vi "LabVIEW host computer v2.0.vi"() -> ()   [LabVIEW 2015]
uses:
  <vilib>/Instr/_visa.llb/VISA Configure Serial Port (Instr).vi
panel:
  out "CH1/CH2":dbl(graph)
  in  "选项卡控件":enum32{"串口配置 ", "数据显示"}(tab)
  in  "VISA resource name":refnum<visa-resource-name> caption="选择串口"
  in  "baud rate (9600)":u32=9600 caption="波特率"
  out "CH1 Power":dbl
  out "?":string
  out "CH2 Power":dbl
  out "?":string
  out "CH1/CH2":dbl format="%#_3g"
  out "当前时间":string
  out "CH2 Power":dbl(graph)
  out "CH1 Power":dbl(graph)
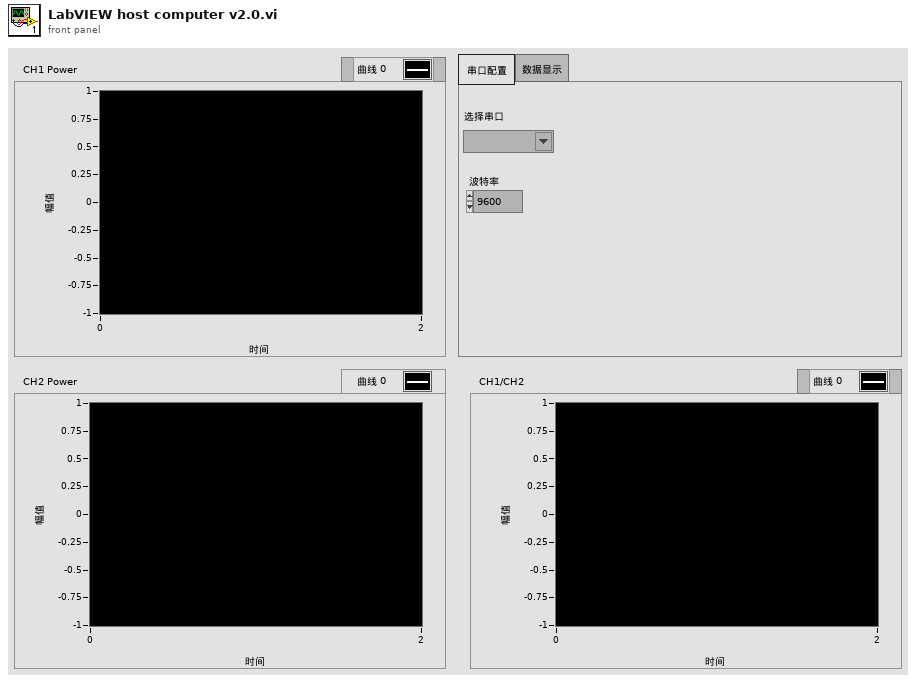
[diagram p1: front panel]
types:
  T1 = enum16{"open", "replace", "create", "open or create", "replace or create", "replace or create with confirmation"}
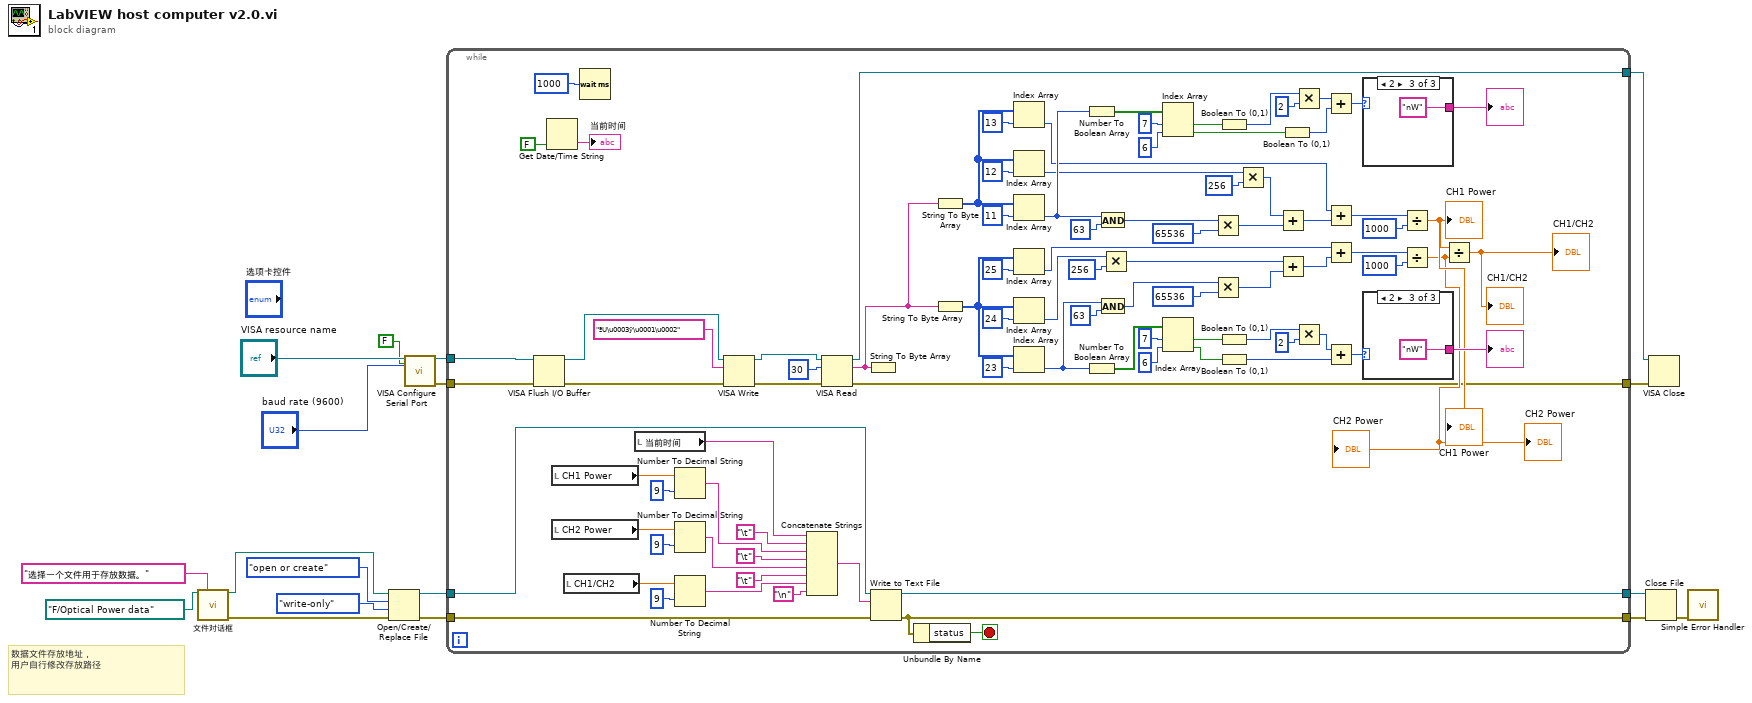
[diagram p0: block diagram]
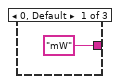
[diagram p2: hidden frame]
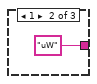
[diagram p3: hidden frame]
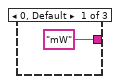
[diagram p4: hidden frame]
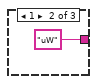
[diagram p5: hidden frame]
diagram:
  # "数据文件存放地址，\n用户自行修改存放路径"
  n1 = call "文件对话框"("start path"=path "F:/Optical Power data", "prompt"="选择一个文件用于存放数据。") -> ("selected path"=w9:path, "error out"=w8:errorcluster)  [unwired: 10 in, 2 out]
  n2 = Open/Create/Replace File(file path (use dialog)=w9, error in=w8, operation (0:open)=T1."open or create" ("操作(0:open)"), access (0:read/write)=enum16{"read/write", "read-only", "write-only"}."write-only" ("权限(0:read/write)")) -> (refnum out=w4:refnum<file>, error out=w5:errorcluster)  [unwired: 2 in, 1 out]
  n3 = call-poly "VISA Configure Serial Port"("VISA resource name"="VISA resource name", "Enable Termination\nChar (T)"=FALSE ("Enable Termination\nChar (T)"), "baud rate (9600)"="baud rate (9600)") -> ("VISA resource name out"=w15:refnum<visa-resource-name>, "error out"=w14:errorcluster)  [unwired: 11 in]
  n4 = while {
    tunnel: w15 -> [w48]
    tunnel: w14 -> [w47]
    tunnel: [w46] -> w13
    tunnel: [w43] -> w12
    tunnel: w5 -> [w41]
    tunnel: w4 -> [w40]
    tunnel: [w31] -> w2
    tunnel: [w33] -> w1
    stop <- w30 stop-if-true
    n5 = VISA Flush I/O Buffer(VISA resource name=w48, error in (no error)=w47) -> (VISA resource name out=w78:refnum<visa-resource-name>, error out=w77:errorcluster)  [unwired: 1 in]
    n6 = Get Date/Time String(want seconds? (F)=FALSE ("需要秒？(F)")) -> (time string=→"当前时间":string)  [unwired: 2 in, 1 out]
    n7 = local read "CH1 Power"() -> (w26:dbl)
    n8 = local read "CH2 Power"() -> (w25:dbl)
    n9 = local read "CH1/CH2"() -> (w24:dbl)
    n10 = Wait (ms)(milliseconds to wait=u32 1000 ("等待时间（毫秒）")) -> ()  [unwired: 1 out]
    n11 = local read "当前时间"() -> (w36:string)
    n12 = Number To Decimal String(number=w26, width (-)=i16 9 ("宽度(-)")) -> (decimal integer string=w23:string)
    n13 = Number To Decimal String(number=w25, width (-)=i16 9 ("宽度(-)")) -> (decimal integer string=w22:string)
    n14 = Number To Decimal String(number=w24, width (-)=i16 9 ("宽度(-)")) -> (decimal integer string=w19:string)
    n15 = VISA Write(VISA resource name=w78, write buffer="ªU\u0003ÿ\u0001\u0002" ("写入缓冲区"), error in (no error)=w77) -> (VISA resource name out=w108:refnum<visa-resource-name>, error out=w107:errorcluster)  [unwired: 1 out]
    n16 = Concatenate Strings(w36, "\t", w23, "\t", w22, "\t", w19, "\n") -> (w32:string)
    n17 = VISA Read(VISA resource name=w108, byte count=u32 30 ("字节总数"), error in (no error)=w107) -> (VISA resource name out=w46:refnum<visa-resource-name>, read buffer=w49:string, error out=w43:errorcluster)  [unwired: 1 out]
    n18 = String To Byte Array(string=w49) -> ()  [unwired: 1 out]
    n19 = Write to Text File(file (use dialog)=w40, text=w32, error in=w41) -> (refnum out=w33:refnum<file>, error out=w31:errorcluster)  [unwired: 1 in, 1 out]
    n20 = Unbundle By Name(w31) -> ("status"=w30:bool)
    n21 = String To Byte Array(string=w49) -> (unsigned byte array=w104:u8[])
    n22 = String To Byte Array(string=w49) -> (unsigned byte array=w75:u8[])
    n23 = Index Array(array=w104, index=13) -> (element=w89:u8)
    n24 = Index Array(array=w104, index=12) -> (element=w95:u8)
    n25 = Index Array(array=w104, index=11) -> (element=w101:u8)
    n26 = Index Array(array=w75, index=25) -> (element=w60:u8)
    n27 = Index Array(array=w75, index=24) -> (element=w66:u8)
    n28 = Index Array(array=w75, index=23) -> (element=w72:u8)
    n29 = Number To Boolean Array(number=w101) -> (Boolean array=w102:bool[])
    n30 = Number To Boolean Array(number=w72) -> (Boolean array=w73:bool[])
    n31 = And(x=w101, y=63) -> (x .and. y?=w93:i32)
    n32 = And(x=w72, y=63) -> (x .and. y?=w64:i32)
    n33 = Multiply(x=w66, y=u32 256) -> (x*y=w68:u32)
    n34 = Index Array(array=w102, index #1=7 ("index"), index #2=6 ("索引")) -> (element #1=w87:bool, element #2=w85:bool)
    n35 = Index Array(array=w73, index #1=7 ("index"), index #2=6 ("索引")) -> (element #1=w58:bool, element #2=w56:bool)
    n36 = Multiply(x=w93, y=u32 65536) -> (x*y=w98:u32)
    n37 = Multiply(x=w64, y=u32 65536) -> (x*y=w69:u32)
    n38 = Boolean To (0,1)(Boolean=w87) -> (0, 1=w86:i16)
    n39 = Boolean To (0,1)(Boolean=w58) -> (0, 1=w57:i16)
    n40 = Boolean To (0,1)(Boolean=w56) -> (0, 1=w53:i16)
    n41 = Multiply(x=w95, y=u32 256) -> (x*y=w97:u32)
    n42 = Add(x=w97, y=w98) -> (x+y=w99:u32)
    n43 = Add(x=w68, y=w69) -> (x+y=w70:u32)
    n44 = Boolean To (0,1)(Boolean=w85) -> (0, 1=w82:i16)
    n45 = Multiply(x=w86, y=2 ("index")) -> (x*y=w83:i32)
    n46 = Multiply(x=w57, y=2 ("index")) -> (x*y=w54:i32)
    n47 = Add(x=w83, y=w82) -> (x+y=w81:i32)
    n48 = Add(x=w89, y=w99) -> (x+y=w80:u32)
    n49 = Add(x=w60, y=w70) -> (x+y=w51:u32)
    n50 = Add(x=w54, y=w53) -> (x+y=w52:i32)
    n51 = case shown="2" w81 {
      tunnel: ["mW" "uW" "nW"] -> w79
      frame 0, Default {
      }
      frame 1 {
      }
      frame 2 {
      }
    }
    "?" <- w79
    n52 = case shown="2" w52 {
      tunnel: ["mW" "uW" "nW"] -> w50
      frame 0, Default {
      }
      frame 1 {
      }
      frame 2 {
      }
    }
    "?" <- w50
    n53 = Divide(x=w80, y=u32 1000) -> (x/y=w45:dbl)
    "CH1 Power" <- w45
    "CH1 Power" <- w45
    n54 = Divide(x=w51, y=u32 1000) -> (x/y=w44:dbl)
    "CH2 Power" <- w44
    "CH2 Power" <- w44
    n55 = Divide(x=w45, y=w44) -> (x/y=→"CH1/CH2" →"CH1/CH2":dbl)
  }
  n56 = Close File(refnum=w1, error in=w2) -> (error out=w3:errorcluster)  [unwired: 1 out]
  n57 = VISA Close(VISA resource name=w13, error in (no error)=w12) -> ()  [unwired: 1 out]
  n58 = call <vilib>:"Simple Error Handler.vi"("error in (no error)"=w3) -> ()  [unwired: 4 in, 5 out]
